vi "TDMS Write with Buffer Prop.vi"(7 "Buffer Size":i32=10000, 8 "error in (no error)":errorcluster, 9 "Data":dbl[][](array[numeric]), 10 "Timestamps":timestamp[][](array[timestamp]), 11 "Path":path) -> (0 "error out":errorcluster, 2 "Time for Write (S)":dbl, 3 "Path Out":path)   [LabVIEW 2017, in "labview-standard-library.lvlib"]
doc: "Uses a common method of writing to file that will typically cause fragmentation. That is switching between writing timestamps and writing data channels. This VI includes setting a buffer size to minimise fragmentation"
uses:
  labview-standard-library.lvlib
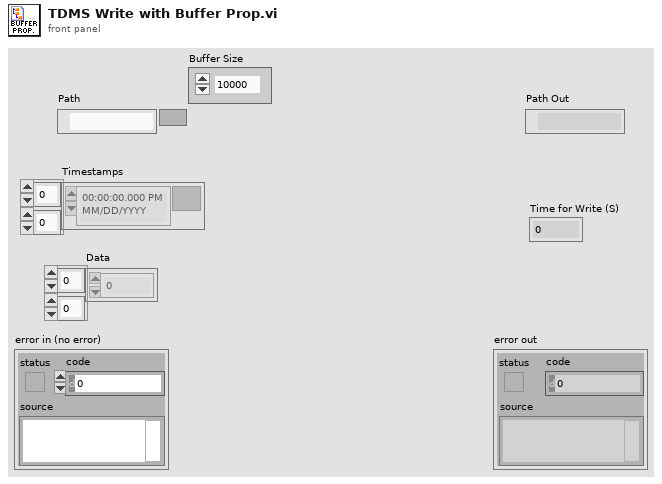
[diagram p1: front panel]
types:
  T1 = enum16{"open", "open or create", "create or replace", "create", "open (read-only)"}
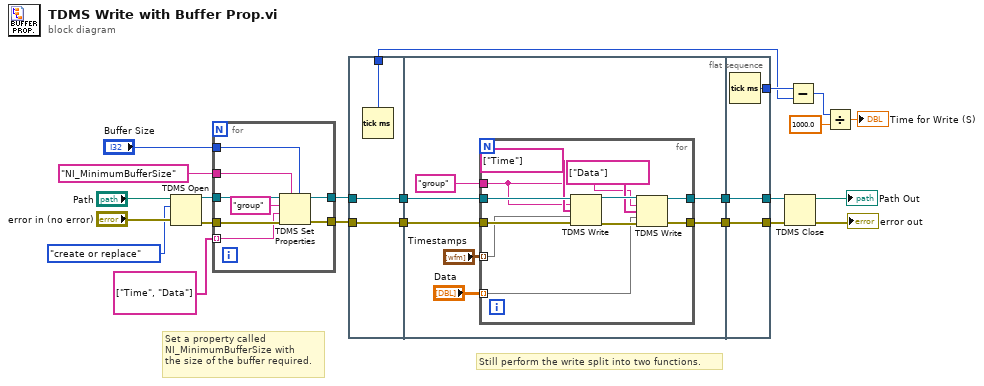
[diagram p0: block diagram]
diagram:
  # "Still perform the write split into two functions."
  # "Set a property called\nNI_MinimumBufferSize with\nthe size of the buffer required."
  n1 = TDMS Open(8:"error in (no error)", 10:T1."create or replace" ("operation (0:open)"), 11:"Path") -> (0:w6:errorcluster, 3:w7:refnum<k34>)  [unwired: 4 in]
  n2 = for {
    tunnel: w7 -> [w31]
    tunnel: w6 -> [w30]
    tunnel: [w29] -> w5
    tunnel: [w28] -> w4
    tunnel: string[] ["Time", "Data"] ("channel name(s) in (Untitled)") -> [w27] mode=indexing
    tunnel: "NI_MinimumBufferSize" -> [w26]
    tunnel: "Buffer Size" -> [w25]
    n3 = TDMS Set Properties(5:w25, 7:w26, 8:w30, 9:w27, 10:"group" ("group name"), 11:w31) -> (0:w28:errorcluster, 3:w29:refnum<k34>)  [unwired: 2 out]
  }
  n4 = flat-sequence {
    tunnel: [w34] -> w21
    tunnel: w5 -> [w34]
    tunnel: [w33] -> w20
    tunnel: w4 -> [w33]
    tunnel: [w32] -> w12
    tunnel: w21 -> [w39]
    tunnel: w20 -> [w38]
    tunnel: [w37] -> w15
    tunnel: [w36] -> w14
    tunnel: [w54] -> w18
    tunnel: [w55] -> w19
    tunnel: w15 -> [w55]
    tunnel: w14 -> [w54]
    tunnel: [w53] -> w13
    frame #0 {
      n5 = Tick Count (ms)() -> (millisecond timer value=w32:u32)
    }
    frame #1 {
      n6 = for {
        tunnel: "Timestamps" -> [w46] mode=indexing
        tunnel: "Data" -> [w45] mode=indexing
        tunnel: w39 -> [w52]
        tunnel: w38 -> [w51]
        tunnel: [w44] -> w37
        tunnel: [w43] -> w36
        tunnel: "group" ("group name") -> [w42]
        n7 = TDMS Write(0:w52, 5:w42, 7:string[] ["Time"] ("channel name(s) in (Untitled)"), 9:w46, 11:w51) -> (4:w50:refnum<k34>, 15:w49:errorcluster)  [unwired: 1 in, 2 out]
        n8 = TDMS Write(0:w50, 5:w42, 7:string[] ["Data"] ("channel name(s) in (Untitled)"), 9:w45, 11:w49) -> (4:w44:refnum<k34>, 15:w43:errorcluster)  [unwired: 1 in, 2 out]
      }
    }
    frame #2 {
      n9 = Tick Count (ms)() -> (millisecond timer value=w53:u32)
    }
  }
  n10 = TDMS Close(8:w18, 11:w19) -> (0:→"error out":errorcluster, 3:→"Path Out":path)
  n11 = Subtract(x=w13, y=w12) -> (x-y=w11:u32)
  n12 = Divide(x=w11, y=1000.0) -> (x/y=→"Time for Write (S)":dbl)
